vi "Constants.vi"() -> ()   [LabVIEW 2019, in "Software Multi-Plex Shared.lvlib"]
doc: "Use this Global VI to access the GUIDs assigned to the page resources of the Custom Device."
uses:
  Software Multi-Plex Shared.lvlib
panel:
  in  "Tab Control":enum32{"GUIDS", "Constants", "Properties"}(tab)
  in  "GUID::Input 3":string="bb107371-342f-4e74-a729-9a180c7afd87"
  in  "GUID::Output":string="dd786ee9-856f-42b8-938b-ea7d801d6c35"
  in  "GUID::Input 2":string="b828d39d-a370-4ba9-a2f2-e646931ac0d5"
  in  "GUID::Input 1":string="9f18dc13-e592-4b02-ba31-c3f4df680c59"
  in  "GUID::Selector":string="f771f13a-6075-4c4a-afb5-40bc181a976f"
  in  "GUID::Channel":string="cd82092f-74ab-4110-acf8-fe4599a5dcd2"
  in  "GUID::Software Multi-Plex":string="8413aea8-b960-4338-8def-49dbabb5ab11"
  in  "Prop::Output Path":string="OutputPath"
  in  "Prop::Input Path":string="InputPath"
  in  "Prop::Compiled.Settings":string="Compiled.Settings"
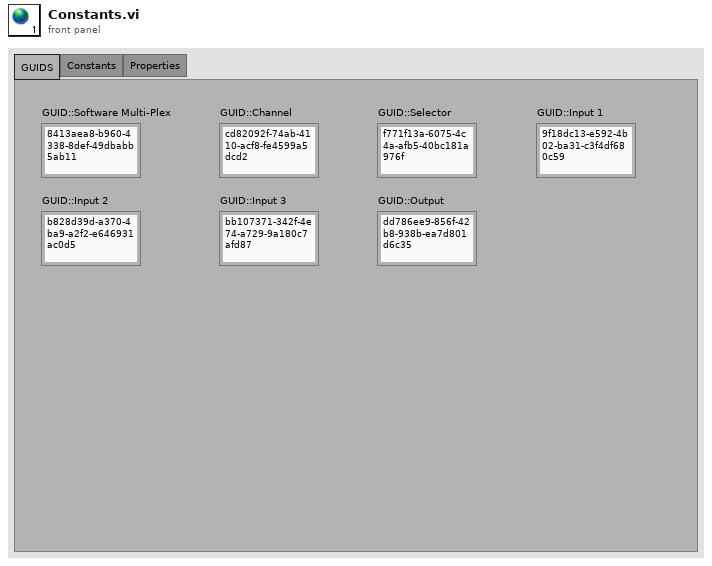
[diagram p1: front panel]
diagram:
